vi "Event_touch_possesion.vi"(8 "error in (no error)":errorcluster, 10 "Game in":refnum<class "Game.lvclass">, 11 "Events in":refnum<class "Events.lvclass">) -> (0 "error out":errorcluster, 3 "Events out":refnum<class "Events.lvclass">)   [LabVIEW 2018, in "Events.lvclass"]
uses:
  Events.lvclass
  Game_class/Game.lvclass
  Game_class/Game.lvclass/Game.ctl
  Team_class/Team.lvclass/Team.ctl
  Object_class/Object.lvclass/Object.ctl
  Parameters_class/Parameters.lvclass/Parameters.ctl
  Robot_class/Robot.lvclass/Robot.ctl
  Events.lvclass/Events.ctl
  <vilib>/Analysis/coordinate.llb/Wrap Angle (scalar).vi
  Object_class/Read x.vi
  Object_class/Read y.vi
  Robot_class/Read orientation.vi
  Robot_class/Read id.vi
  <vilib>/Analysis/_algsub.llb/Real Vector Norm.vi
  Game_class/Read AllyRef.vi
  Game_class/Read EnemyRef.vi
  Game_class/Read BallRef.vi
  Game_class/Read Parameters.lvclass.vi
  Game_class/Read Utilities.lvclass.vi
  Parameters_class/Read DistanceForPossession.vi
  Parameters_class/Read AngularToleranceForPossession.vi
  Parameters_class/Read TouchDistance.vi
  Parameters_class/Read DistanceForaStillBall.vi
  Team_class/Read RobotRef.vi
  Write id_touch.vi
  Write enemy_ball_possesion.vi
  Write id_enemy_ball_possesion.vi
  Write our_balll_possesion.vi
  Write id_our_balll_possesion.vi
  Write touch.vi
  Ball_class/Ball.lvclass
  C:/Users/Leonardo/Documents/RoboIme/Futebol/SSL/SSL-Phoenix/SSL_AI/Object_class/Object.lvclass
  Enemy_class/Enemy.lvclass
  C:/Users/Leonardo/Documents/RoboIme/Futebol/SSL/SSL-Phoenix/SSL_AI/Team_class/Team.lvclass
  Ally_class/Ally.lvclass
  Robot_class/Robot.lvclass
  Parameters_class/Parameters.lvclass
  Utilities_class/Utilities.lvclass
  <vilib>/Analysis/NI_AAL_Angle.lvlib
  <vilib>/Analysis/NI_AALPro.lvlib
panel:
  out "id possesion":dbl
  out "Our Possession":bool
  out "id enemy possesion":dbl
  out "enemy_ball_possession":bool
  out "id touch":dbl
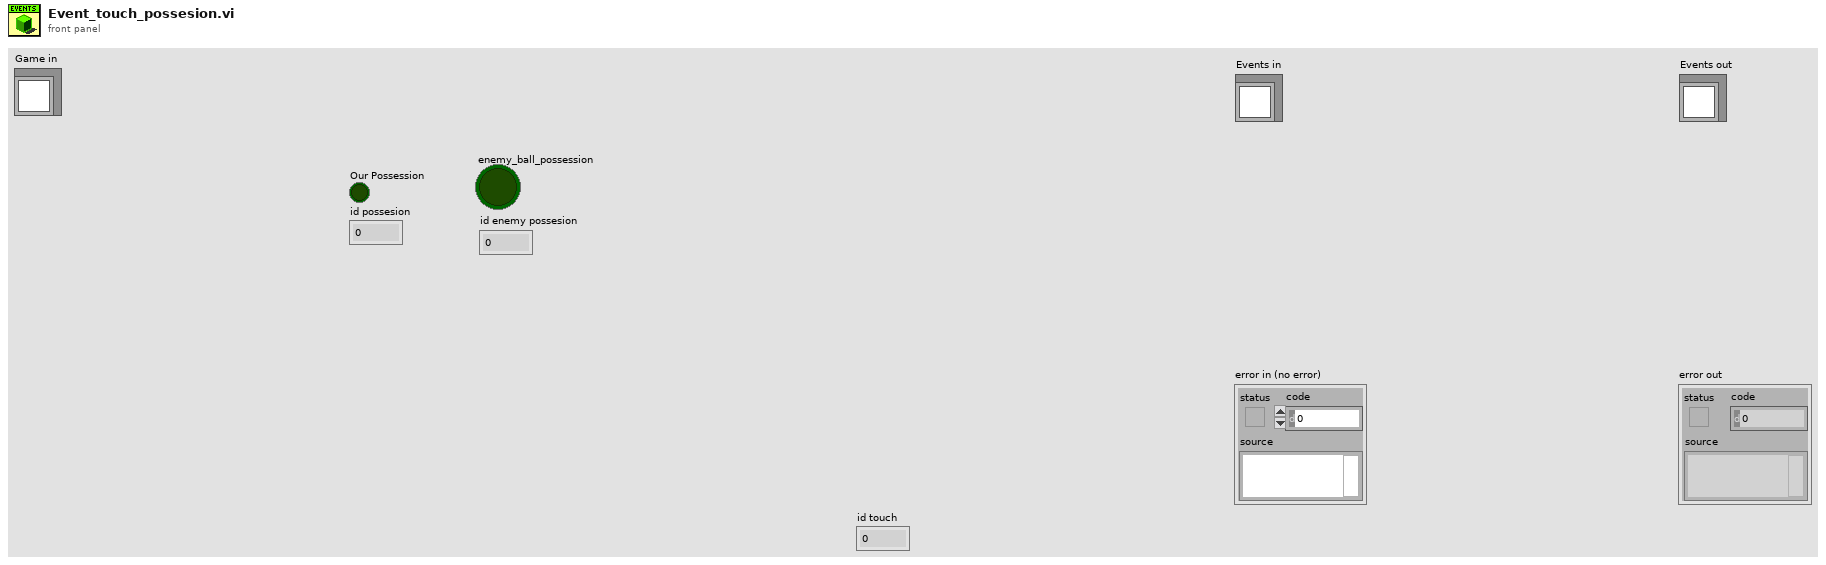
[diagram p1: front panel]
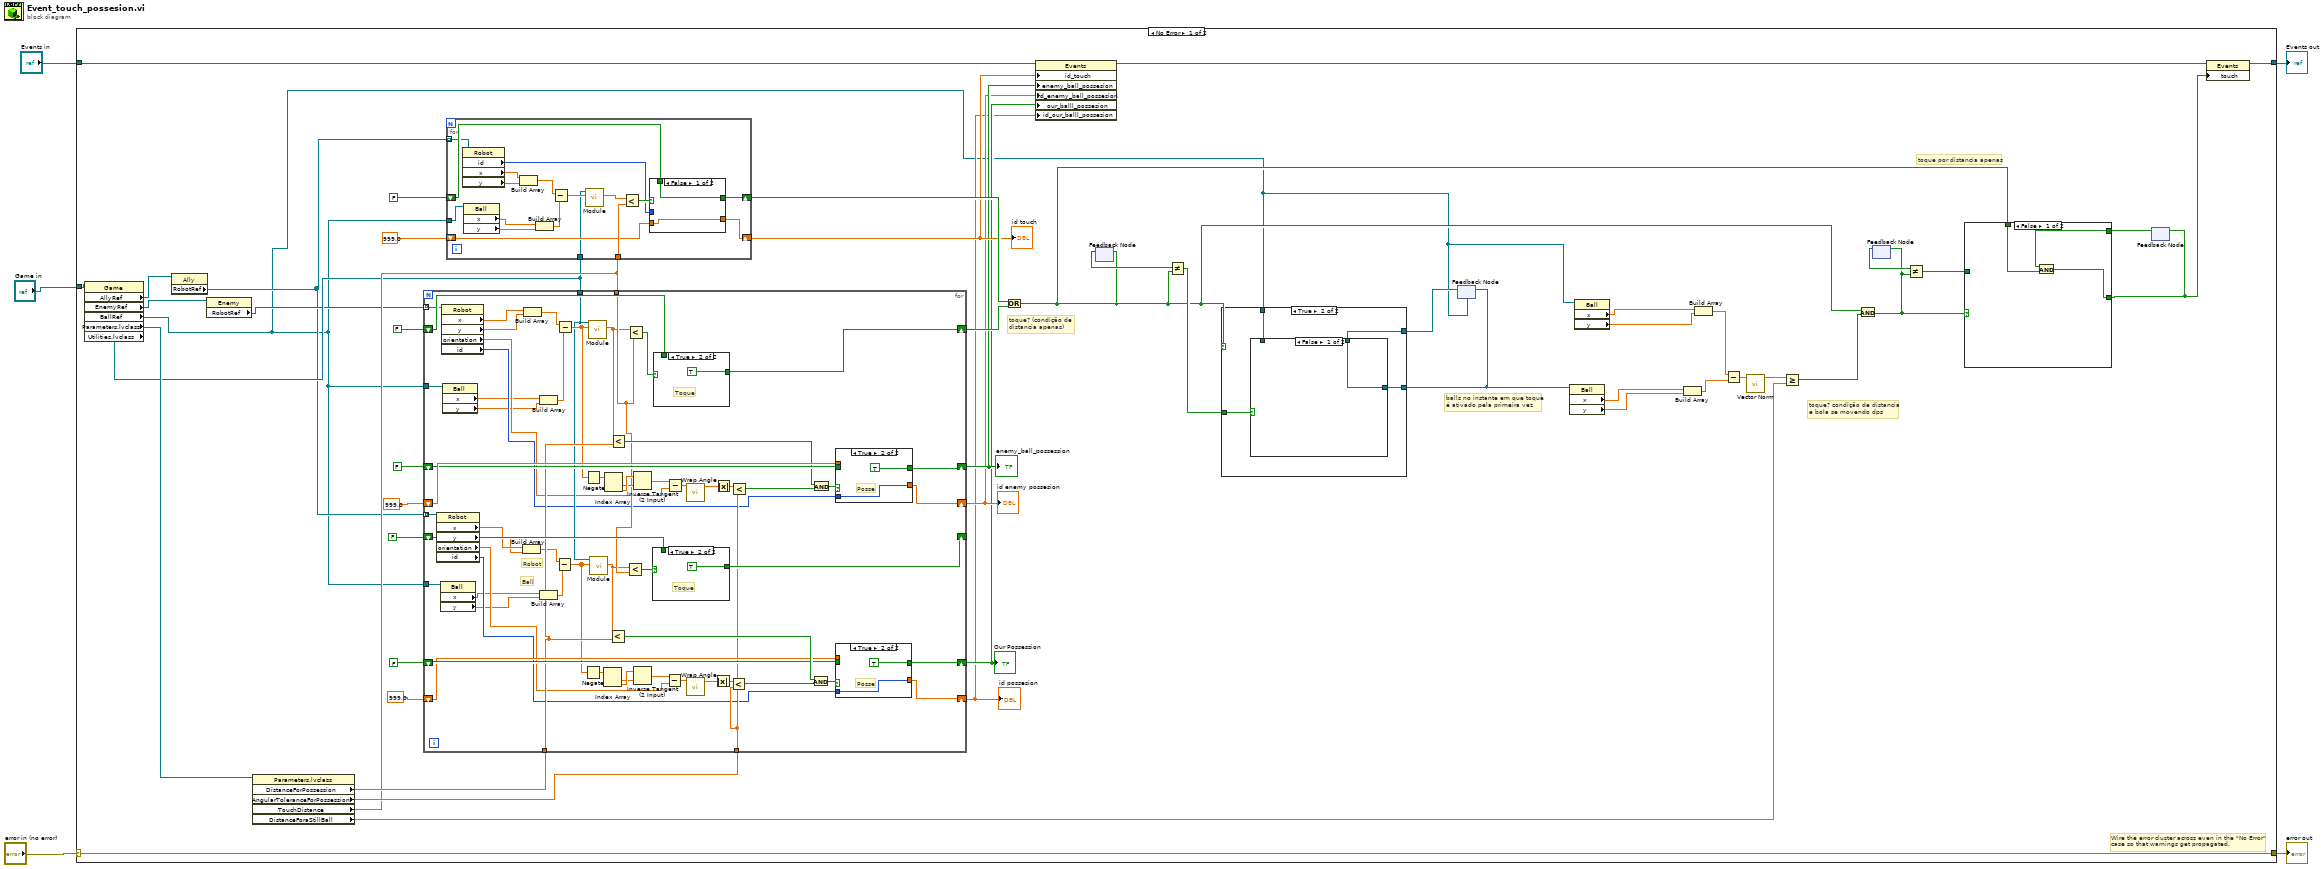
[diagram p0: block diagram]
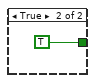
[diagram p3: hidden frame]
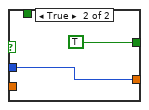
[diagram p10: hidden frame]
diagram:
  n1 = case shown="No Error" "error in (no error)" {
    selector: "error in (no error)" -> [w55 w168]
    tunnel: [w55 w168] -> w4
    tunnel: [w24 w167] -> w2
    tunnel: "Events in" -> [w31 w167]
    tunnel: "Game in" -> [w19 _]
    frame No Error {
      # "toque por distancia apenas"
      # "toque? condição de distancia\ne bola se movendo dps"
      # "balls no instante em que toque\né ativado pela primeira vez"
      # "toque? (condição de \ndistancia apenas)"
      # "Wire the error cluster across even in the \"No Error\"\ncase so that warnings get propagated."
      n2 = property class="Game"(reference=w19) -> ("AllyRef"=w17:refnum<class "Ally.lvclass">, "EnemyRef"=w14:refnum<class "Enemy.lvclass">, "BallRef"=w11:refnum<class "Ball.lvclass">, "Parameters.lvclass"=w16:refnum<class "Parameters.lvclass">, "Utilities.lvclass"=w15:refnum<class "Utilities.lvclass">)  [unwired: 1 in, 2 out]
      n3 = property class="Ally"(reference=w17) -> ("RobotRef"=w12:refnum<class "Robot.lvclass">[])  [unwired: 1 in, 2 out]
      n4 = property class="Enemy"(reference=w14) -> ("RobotRef"=w13:refnum<class "Robot.lvclass">[])  [unwired: 1 in, 2 out]
      n5 = property class="Parameters.lvclass"(reference=w16) -> ("DistanceForPossession"=w22:dbl, "AngularToleranceForPossession"=w21:dbl, "TouchDistance"=w20:dbl, "DistanceForaStillBall"=w18:dbl)  [unwired: 1 in, 2 out]
      n6 = for {
        shift-right: [w129] -> w52
        shift-left: FALSE -> [w128]
        tunnel: w20 -> [w95]
        tunnel: w21 -> [w93]
        shift-right: [w114] -> w28
        shift-left: 999.0 -> [w119]
        tunnel: w22 -> [w94]
        shift-right: [w118] -> w29
        shift-left: FALSE -> [w117]
        shift-right: [w100] -> _
        shift-left: FALSE -> [w101]
        shift-right: [w96] -> w27
        shift-left: FALSE -> [w99]
        shift-right: [w97] -> w26
        shift-left: 999.0 -> [w98]
        tunnel: w15 -> [w88]
        tunnel: w13 -> [w83] mode=indexing
        tunnel: w11 -> [w82]
        tunnel: w12 -> [w75] mode=indexing
        tunnel: w11 -> [w74]
        # "Ball"
        # "Robot"
        n7 = property class="Robot"(reference=w75) -> ("x"=w79:dbl, "y"=w78:dbl, "orientation"=w77:dbl, "id"=w76:i32)  [unwired: 1 in, 2 out]
        n8 = property class="Ball"(reference=w74) -> ("x"=w73:dbl, "y"=w72:dbl)  [unwired: 1 in, 2 out]
        n9 = property class="Robot"(reference=w83) -> ("x"=w87:dbl, "y"=w86:dbl, "orientation"=w85:dbl, "id"=w84:i32)  [unwired: 1 in, 2 out]
        n10 = property class="Ball"(reference=w82) -> ("x"=w81:dbl, "y"=w80:dbl)  [unwired: 1 in, 2 out]
        n11 = Build Array(w79, w78) -> (w71:dbl[])
        n12 = Build Array(w87, w86) -> (w132:dbl[])
        n13 = Build Array(w73, w72) -> (w113:dbl[])
        n14 = Build Array(w81, w80) -> (w131:dbl[])
        n15 = Subtract(x=w71, y=w113) -> (x-y=w90:dbl[])
        n16 = Subtract(x=w132, y=w131) -> (x-y=w92:dbl[])
        n17 = Negate(x=w90) -> (-x=w111:dbl[])
        n18 = Negate(x=w92) -> (-x=w127:dbl[])
        n19 = call-dynamic "Module.vi"("2D vector"=w92, "Utilities in"=w88) -> ("Modulo"=w91:dbl)  [unwired: 7 in, 2 out]
        n20 = call-dynamic "Module.vi"("2D vector"=w90, "Utilities in"=w88) -> ("Modulo"=w89:dbl)  [unwired: 7 in, 2 out]
        n21 = Index Array(array=w111) -> (element #1=w109:dbl, element #2=w110:dbl)  [unwired: 2 in]
        n22 = Index Array(array=w127) -> (element #1=w125:dbl, element #2=w126:dbl)  [unwired: 2 in]
        n23 = Less?(x=w89, y=w94) -> (x < y?=w102:bool)
        n24 = Less?(x=w91, y=w94) -> (x < y?=w115:bool)
        n25 = Less?(x=w89, y=w95) -> (x < y?=w112:bool)
        n26 = Less?(x=w91, y=w95) -> (x < y?=w130:bool)
        n27 = Inverse Tangent (2 Input)(1:w109, 2:w110) -> (0:w108:dbl)
        n28 = Inverse Tangent (2 Input)(1:w125, 2:w126) -> (0:w124:dbl)
        n29 = case shown="True" w112 {
          tunnel: [w137 TRUE] -> w100
          tunnel: w101 -> [w137 _]
          frame False {
            # "Sem toque"
          }
          frame True {
            # "Toque"
          }
        }
        n30 = case shown="True" w130 {
          tunnel: [w143 TRUE] -> w129
          tunnel: w128 -> [w143 _]
          frame False {
            # "Sem toque"
          }
          frame True {
            # "Toque"
          }
        }
        n31 = Subtract(x=w108, y=w77) -> (x-y=w107:dbl)
        n32 = Subtract(x=w124, y=w85) -> (x-y=w123:dbl)
        n33 = call-poly <vilib>:"Wrap Angle.vi"("angle in"=w123) -> ("angle out"=w121:dbl)  [unwired: 9 in, 1 out]
        n34 = call-poly <vilib>:"Wrap Angle.vi"("angle in"=w107) -> ("angle out"=w105:dbl)  [unwired: 9 in, 1 out]
        n35 = Absolute Value(x=w105) -> (abs(x)=w106:dbl)
        n36 = Absolute Value(x=w121) -> (abs(x)=w122:dbl)
        n37 = Less?(x=w106, y=w93) -> (x < y?=w103:bool)
        n38 = Less?(x=w122, y=w93) -> (x < y?=w116:bool)
        n39 = And(x=w102, y=w103) -> (x .and. y?=w104:bool)
        n40 = And(x=w115, y=w116) -> (x .and. y?=w120:bool)
        n41 = case shown="True" w104 {
          tunnel: [w133 TRUE] -> w96
          tunnel: w76 -> [_ w135]
          tunnel: [w134 w135] -> w97
          tunnel: w98 -> [w134 _]
          tunnel: w99 -> [w133 _]
          frame False {
            # "Sem toque"
          }
          frame True {
            # "Posse"
          }
        }
        n42 = case shown="True" w120 {
          tunnel: [w139 TRUE] -> w118
          tunnel: w84 -> [_ w141]
          tunnel: [w140 w141] -> w114
          tunnel: w119 -> [w140 _]
          tunnel: w117 -> [w139 _]
          frame False {
            # "Sem toque"
          }
          frame True {
            # "Posse"
          }
        }
      }
      "enemy_ball_possession" <- w29
      "id enemy possesion" <- w28
      "Our Possession" <- w27
      "id possesion" <- w26
      n43 = for {
        shift-right: [w159] -> w53
        shift-left: FALSE -> [w158]
        tunnel: w20 -> [w157]
        shift-right: [w156] -> w30
        shift-left: 999.0 ("id") -> [w155]
        tunnel: w12 -> [w154] mode=indexing
        tunnel: w11 -> [w150]
        tunnel: w15 -> [w145]
        n44 = property class="Robot"(reference=w154) -> ("id"=w153:i32, "x"=w152:dbl, "y"=w151:dbl)  [unwired: 1 in, 2 out]
        n45 = property class="Ball"(reference=w150) -> ("x"=w149:dbl, "y"=w148:dbl)  [unwired: 1 in, 2 out]
        n46 = Build Array(w152, w151) -> (w162:dbl[])
        n47 = Build Array(w149, w148) -> (w161:dbl[])
        n48 = Subtract(x=w162, y=w161) -> (x-y=w147:dbl[])
        n49 = call-dynamic "Module.vi"("2D vector"=w147, "Utilities in"=w145) -> ("Modulo"=w146:dbl)  [unwired: 7 in, 2 out]
        n50 = Less?(x=w146, y=w157) -> (x < y?=w160:bool)
        n51 = case shown="False" w160 {
          tunnel: [w164 TRUE] -> w159
          tunnel: w158 -> [w164 _]
          tunnel: [w163 w165] -> w156
          tunnel: w153 -> [_ w165]
          tunnel: w155 -> [w163 _]
          frame False {
          }
          frame True {
          }
        }
      }
      "id touch" <- w30
      n52 = Or(x=w53, y=w52) -> (x .or. y?=w33:bool)
      n53 = property class="Events"(reference=w31, "id_touch"=w30, "enemy_ball_possesion"=w29, "id_enemy_ball_possesion"=w28, "our_balll_possesion"=w27, "id_our_balll_possesion"=w26) -> (reference out=w25:refnum<class "Events.lvclass">)  [unwired: 1 in, 1 out]
      n54 = feedback #1() -> (w44:bool)  [unwired: 1 in]
      n55 = feedback-in #1(w33) -> ()
      n56 = Not Equal?(x=w44, y=w33) -> (x != y?=w43:bool)
      n57 = feedback #2(w11) -> (w42:refnum<class "Ball.lvclass">)
      n58 = case shown="True" w33 {
        tunnel: w11 -> [_ w65]
        tunnel: [w64 w67] -> w8
        tunnel: w43 -> [_ w68]
        tunnel: w42 -> [w64 w66]
        frame False {
        }
        frame True {
          n59 = case shown="False" w68 {
            tunnel: [w69 w70] -> w67
            tunnel: w66 -> [w69 _]
            tunnel: w65 -> [_ w70]
            frame False {
            }
            frame True {
            }
          }
        }
      }
      n60 = feedback-in #2(w8) -> ()
      n61 = property class="Ball"(reference=w8) -> ("x"=w7:dbl, "y"=w6:dbl)  [unwired: 1 in, 2 out]
      n62 = property class="Ball"(reference=w11) -> ("x"=w10:dbl, "y"=w9:dbl)  [unwired: 1 in, 2 out]
      n63 = Build Array(w7, w6) -> (w40:dbl[])
      n64 = Build Array(w10, w9) -> (w41:dbl[])
      n65 = Subtract(x=w41, y=w40) -> (x-y=w39:dbl[])
      n66 = call-poly <vilib>:"Vector Norm.vi"("Input Vector"=w39) -> ("norm"=w38:dbl)  [unwired: 9 in, 1 out]
      n67 = Greater Or Equal?(x=w38, y=w18) -> (x >= y?=w37:bool)
      n68 = And(x=w33, y=w37) -> (x .and. y?=w32:bool)
      n69 = feedback #3() -> (w36:bool)  [unwired: 1 in]
      n70 = feedback-in #3(w32) -> ()
      n71 = Not Equal?(x=w36, y=w32) -> (x != y?=w35:bool)
      n72 = feedback #4() -> (w34:bool)  [unwired: 1 in]
      n73 = case shown="False" w32 {
        tunnel: w35 -> [_ w61]
        tunnel: [w56 w60] -> w23
        tunnel: w34 -> [w57 w59]
        tunnel: w33 -> [w58 _]
        frame False {
          n74 = And(x=w57, y=w58) -> (x .and. y?=w56:bool)
        }
        frame True {
          n75 = case shown="False" w61 {
            tunnel: [w62 TRUE] -> w60
            tunnel: w59 -> [w62 _]
            frame False {
            }
            frame True {
            }
          }
        }
      }
      n76 = feedback-in #4(w23) -> ()
      n77 = property class="Events"(reference=w25, "touch"=w23) -> (reference out=w24:refnum<class "Events.lvclass">)  [unwired: 1 in, 1 out]
    }
    frame Error {
    }
  }
  "error out" <- w4
  "Events out" <- w2
